vi "Read One Non-Blank Line.vi"(0 "refnum":refnum<file>, 1 "error in (not an error)":errorcluster) -> (2 "dup refnum":refnum<file>, 3 "Line":string, 4 "error out":errorcluster)   [LabVIEW 2012]
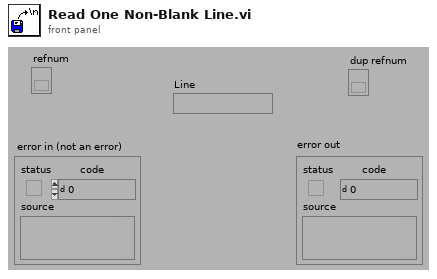
[diagram p1: front panel]
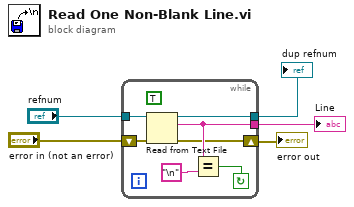
[diagram p0: block diagram]
diagram:
  n1 = while {
    tunnel: [w6] -> w2
    tunnel: [w10] -> w1
    tunnel: "refnum" -> [w11]
    shift-left: "error in (not an error)" -> [w12]
    shift-right: [w7] -> w3
    stop <- w8 continue-if-true
    (unwired) TRUE ("line mode (F)")
    n2 = Read from Text File(file (use dialog)=w11, error in=w12) -> (refnum out=w6:refnum<file>, text=w10:string, error out=w7:errorcluster)  [unwired: 2 in, 1 out]
    n3 = Equal?(x=w10, y="\n") -> (x = y?=w8:bool)
  }
  "error out" <- w3
  "dup refnum" <- w2
  "Line" <- w1
